vi "read json text array  from json text.vi"(8 "error in (no error)":errorcluster, 9 "this vis path":path, 11 "file name":path) -> (0 "error out":errorcluster, 3 "Array out":string[](array[string]))   [LabVIEW 2020]
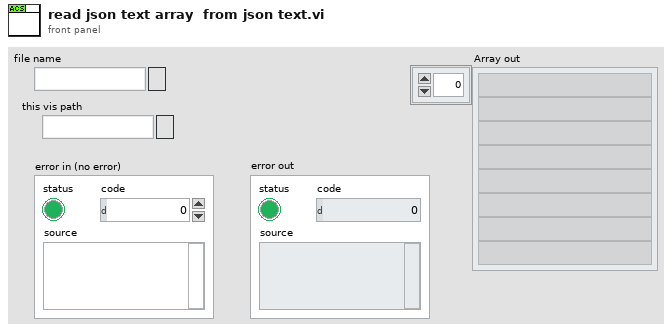
[diagram p1: front panel]
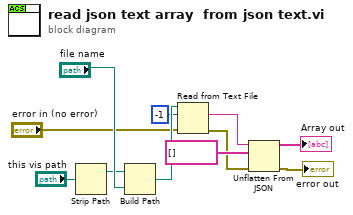
[diagram p0: block diagram]
diagram:
  n1 = Strip Path(path="this vis path") -> (stripped path=w9:path)  [unwired: 1 out]
  n2 = Build Path(base path=w9, name or relative path="file name") -> (appended path=w10:path)
  n3 = Read from Text File(file (use dialog)=w10, count=-1, error in="error in (no error)") -> (text=w6:string, error out=w3:errorcluster)  [unwired: 1 in, 2 out]
  n4 = Unflatten From JSON(JSON string=w6, type and defaults=string[] [], error in (no error)=w3) -> (value=→"Array out":string[], error out=→"error out":errorcluster)  [unwired: 4 in]
